vi "CheckRecordBitFVIR.vi"(11 "Int array data from queue":u16[](array[numeric])) -> (3 "Record bit T/F":bool)   [LabVIEW 2020, in "WritingDataFile.lvlib"]
uses:
  WritingDataFile.lvlib
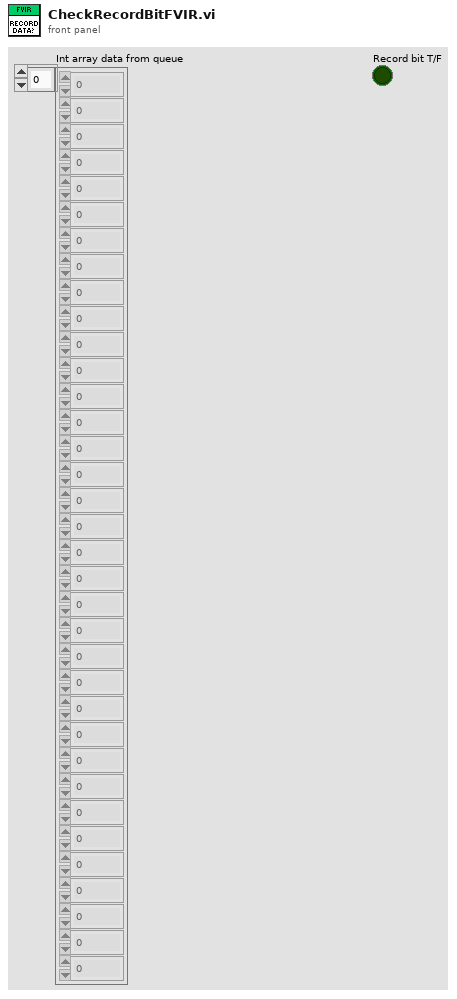
[diagram p1: front panel]
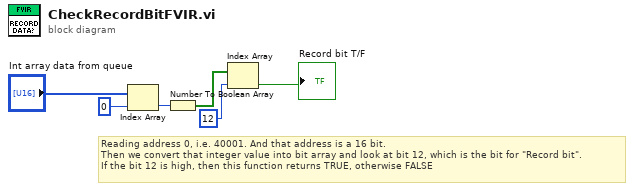
[diagram p0: block diagram]
diagram:
  # "Reading address 0, i.e. 40001. And that address is a 16 bit. \nThen we convert that integer value into bit array and look at bit 12, which is the bit for \"Record bit\". \nIf the bit 12 is high, then this function returns TRUE, otherwise FALSE"
  n1 = Index Array(array="Int array data from queue", index=0) -> (element=w2:u16)
  n2 = Number To Boolean Array(number=w2) -> (Boolean array=w3:bool[])
  n3 = Index Array(array=w3, index=12) -> (element=→"Record bit T/F":bool)
